vi "UMLEditor GettingStartedDialog.vi"   [LabVIEW 2012]
uses:
  <vilib>/Platform/browser.llb/Open URL in Default Browser (path).vi
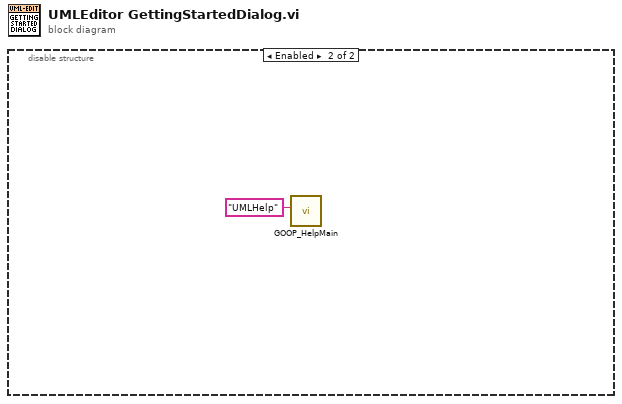
[diagram p0: block diagram]
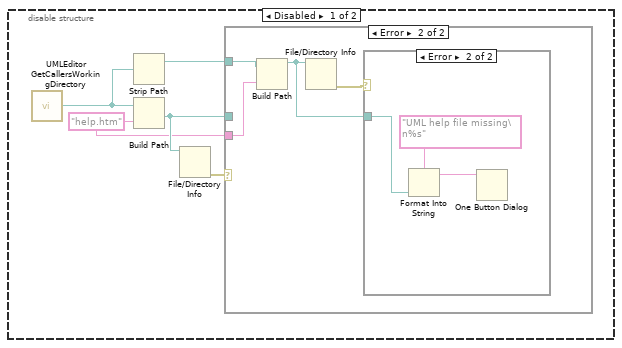
[diagram p2: hidden frame]
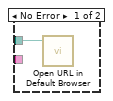
[diagram p3: hidden frame]
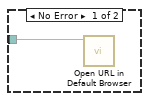
[diagram p4: hidden frame]
diagram:
  n1 = disable-structure shown="Enabled" {
    frame Disabled {
      w1 = "help.htm" ("name or relative path")
      n2 = call <resource>:"UMLEditor GetCallersWorkingDirectory.vi"() -> ("VI directory"=w3:path)  [unwired: 2 in, 9 out]
      n3 = Strip Path(path=w3) -> (stripped path=w2:path)  [unwired: 1 out]
      n4 = Build Path(base path=w3, name or relative path=w1) -> (appended path=w5:path)
      n5 = File/Directory Info(path=w5) -> (error out=w4:errorcluster)  [unwired: 1 in, 6 out]
      n6 = case shown="Error" w4 {
        tunnel: w5 -> [w6 _]
        tunnel: w2 -> [_ w10]
        tunnel: w1 -> [_ w9]
        frame No Error {
          n7 = call-poly <vilib>:"Open URL in Default Browser.vi"("path"=w6) -> ()  [unwired: 1 in, 6 out]
        }
        frame Error {
          n8 = Build Path(base path=w10, name or relative path=w9) -> (appended path=w7:path)
          n9 = File/Directory Info(path=w7) -> (error out=w8:errorcluster)  [unwired: 1 in, 6 out]
          n10 = case shown="Error" w8 {
            tunnel: w7 -> [w11 w14]
            frame No Error {
              n11 = call-poly <vilib>:"Open URL in Default Browser.vi"("path"=w11) -> ()  [unwired: 1 in, 6 out]
            }
            frame Error {
              n12 = Format Into String(format string="UML help file missing\n%s" ("message"), w14) -> (resulting string=w12:string)  [unwired: 2 in, 1 out]
              n13 = One Button Dialog(message=w12) -> ()  [unwired: 2 out]
            }
          }
        }
      }
    }
    frame Enabled {
      n14 = call <resource>:"GOOP_HelpMain.vi"("File"="UMLHelp") -> ()  [unwired: 11 in]
    }
  }
